vi "Start Command.vi"(8 "error in (no error)":errorcluster, 10 "Robot Actors.lvlib:Command.lvlib:Command.lvclass":refnum<class "Command Actor.lvclass">, 11 "No Command in":refnum<class "No Command.lvclass">) -> (0 "error out":errorcluster, 3 "No Command out":refnum<class "No Command.lvclass">)   [LabVIEW 2014, in "Robot Actor Framework.lvlib" / "Command Processor Actor.lvlib" / "No Command.lvclass"]
uses:
  No Command.lvclass
  Command Actor/Command Actor Class/Command Actor.lvclass
  <vilib>/ActorFramework/Message Enqueuer/Message Priority.ctl
  <vilib>/ActorFramework/Actor/Actor.lvclass/Actor.ctl
  <vilib>/ActorFramework/Message Enqueuer/Message Enqueuer.lvclass/Message Enqueuer.ctl
  <vilib>/ActorFramework/Message Enqueuer/Init from Existing Queue.vi
  <vilib>/ActorFramework/Message Enqueuer/Enqueue.vi
  <vilib>/ActorFramework/Message Priority Queue/Priority Enqueue.vi
  Command Processor Actor Class/Command Processor Actor.lvclass
  <vilib>/ActorFramework/Message Enqueuer/Message Enqueuer.lvclass
  Command Processor Actor Messages/Go To Starting Command Msg/Go To Starting Command Msg.lvclass
  <vilib>/ActorFramework/Actor/Actor.lvclass
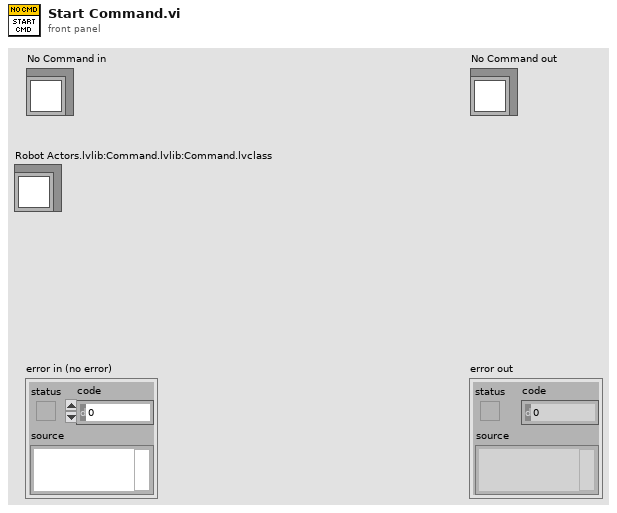
[diagram p1: front panel]
types:
  T1 = typedef "Actor Framework.lvlib/Message Enqueuer.lvclass/Message Priority.ctl" = enum16{"Low", "Normal", "High"}
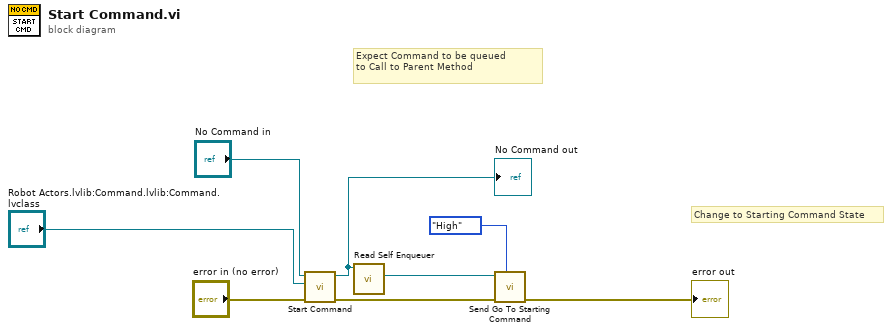
[diagram p0: block diagram]
diagram:
  # "Expect Command to be queued\nto Call to Parent Method"
  # "Change to Starting Command State"
  n1 = call-parent "Start Command.vi"("error in (no error)"="error in (no error)", "Robot Actors.lvlib:Command.lvlib:Command.lvclass"="Robot Actors.lvlib:Command.lvlib:Command.lvclass", "Command Processor in"="No Command in") -> ("error out"=w5:errorcluster, "Command Processor out"=w1:refnum<class "No Command.lvclass">)  [unwired: 7 in]
  "No Command out" <- w1
  n2 = call <vilib>:"Read Self Enqueuer.vi"("Actor"=w1) -> ("Self Enqueuer"=w8:refnum<class "Message Enqueuer.lvclass">)  [unwired: 10 in]
  n3 = call "Send Go To Starting Command.vi"("Message Priority (Normal)"=Message_Priority."High", "error in (no error)"=w5, "Message Enqueuer"=w8) -> ("error out"=→"error out":errorcluster)  [unwired: 7 in, 1 out]
